vi "ma_HasFIRSpecsChanged.vi"(4 "optional FIR filter specifications":T1={"PB Gain"=-3.0, "SB Gain"=-60.0, "Scale"=TRUE, "Window"=enum."Flat Top"} {"SB Gain" format="%0.2f"; "PB Gain" format="%0.2f"}, 6 "FIR Filter Specifications":T2={"Topology"=enum."Off", "Type"=enum."Lowpass", "#Taps"=1, "Lower PB"=100.0, "Upper PB"=200.0, "Lower SB"=1.0, "Upper SB"=60.0} {"Lower SB" format="%0.2p"; "Upper SB" format="%0.2p"; "Lower PB" format="%0.2p"; "Upper PB" format="%0.2p"}, 8 "error in (no error)":errorcluster, 10 "redesign filter":bool) -> (0 "error out":errorcluster, 3 "ValsDifferent?":bool)   [LabVIEW 2020, in "NI_MAPro.lvlib"]
uses:
  NI_MAPro.lvlib
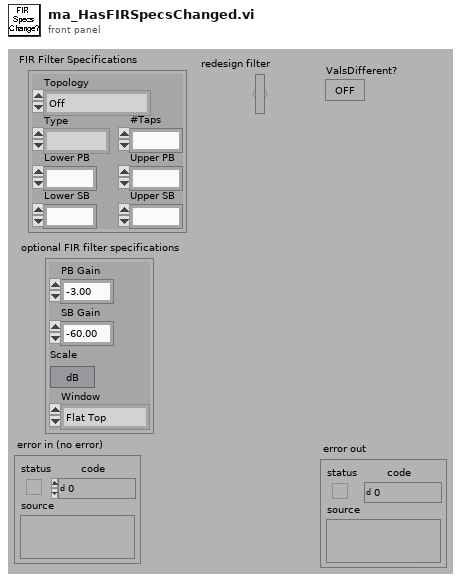
[diagram p1: front panel]
types:
  T1 = cluster{"PB Gain":dbl, "SB Gain":dbl, "Scale":bool, "Window":enum16{"None", "Hanning", "Hamming", "Triangular", "Blackman", "Exact Blackman", "Blackman-Harris", "Kaiser-Bessel", "Flat Top"}}
  T2 = cluster{"Topology":enum16{"Off", "FIR by Specification", "Equi-ripple FIR", "Windowed FIR"}, "Type":enum16{"Lowpass", "Highpass", "Bandpass", "Bandstop"}, "#Taps":i32, "Lower PB":dbl, "Upper PB":dbl, "Lower SB":dbl, "Upper SB":dbl}
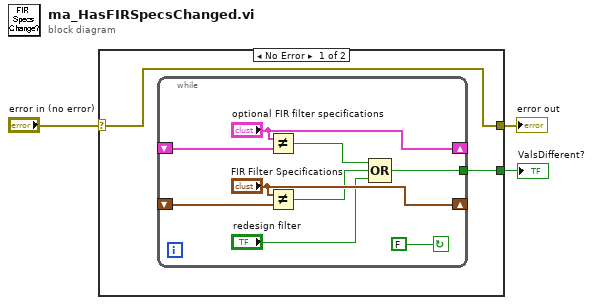
[diagram p0: block diagram]
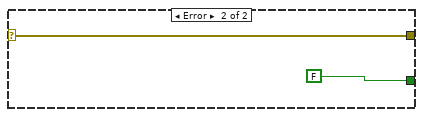
[diagram p2: hidden frame]
diagram:
  n1 = case shown="No Error" "error in (no error)" {
    selector: "error in (no error)" -> [w4 w15]
    tunnel: [w5 FALSE] -> w2
    tunnel: [w4 w15] -> w1
    frame No Error {
      n2 = while {
        shift-left: _ -> [w13]
        shift-right: ["FIR Filter Specifications"] -> _
        tunnel: [w7] -> w5
        shift-left: _ -> [w11]
        shift-right: ["optional FIR filter specifications"] -> _
        stop <- FALSE continue-if-true
        n3 = Not Equal?(x="optional FIR filter specifications", y=w11) -> (x != y?=w9:bool)
        n4 = Not Equal?(x="FIR Filter Specifications", y=w13) -> (x != y?=w8:bool)
        n5 = Compound Arithmetic op=OR(w9, w8, "redesign filter") -> (w7:bool)
      }
    }
    frame Error {
    }
  }
  "error out" <- w1
  "ValsDifferent?" <- w2
